vi "pmu_Compute Phasor Indexes.vi"(8 "error in (no error)":errorcluster, 10 "physical channels":T3[](array[typedef]), 11 "phasor channels":T2[](array[typedef]) {"phasor unit scaling" max=16777215 format="%06x"; "phasor unit" items=["Voltage [V]"=0, "Current [A]"=16777216]}) -> (0 "error out":errorcluster, 3 "phasor channel info":T1[](array[typedef]))   [LabVIEW 2011, in "NI_EP_PMU.lvlib"]
uses:
  <vilib>/addons/Electrical Power/PMU/NI_EP_PMU.lvlib
  <vilib>/addons/Electrical Power/PMU/Common/Controls/pmu_Physical Channel.ctl
  <vilib>/addons/Electrical Power/PMU/Common/Controls/pmu_Channel Phase.ctl
  <vilib>/addons/Electrical Power/PMU/Common/Controls/pmu_Phasor Channel.ctl
  <vilib>/addons/Electrical Power/PMU/Common/Controls/pmu_Phasor Channel Info.ctl
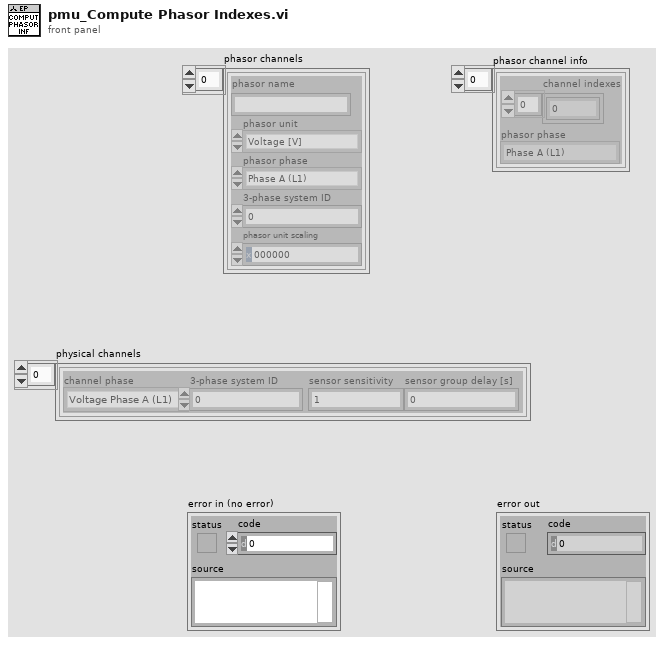
[diagram p1: front panel]
types:
  T1 = typedef "NI_EP_PMU.lvlib/pmu_Phasor Channel Info.ctl" = cluster{"channel indexes":i32[], "phasor phase":enum16{"Phase A (L1)", "Phase B (L2)", "Phase C (L3)", "Phase N", "Positive sequence", "Negative sequence", "Zero sequence"}}
  T2 = typedef "NI_EP_PMU.lvlib/pmu_Phasor Channel.ctl" = cluster{"phasor name":string, "phasor unit":u32, "phasor phase":enum16{"Phase A (L1)", "Phase B (L2)", "Phase C (L3)", "Phase N", "Positive sequence", "Negative sequence", "Zero sequence"}, "3-phase system ID":u8, "phasor unit scaling":u32}
  T3 = typedef "NI_EP_PMU.lvlib/pmu_Physical Channel.ctl" = cluster{"channel phase":T4, "3-phase system ID":u8, "sensor sensitivity":dbl, "sensor group delay [s]":dbl}
  T4 = typedef "NI_EP_PMU.lvlib/pmu_Channel Phase.ctl" = enum16{"Voltage Phase A (L1)", "Voltage Phase B (L2)", "Voltage Phase C (L3)", "Voltage Phase N (Neutral)", "Current Phase A (L1)", "Current Phase B (L2)", "Current Phase C (L3)", "Current Phase N (Neutral)"}
  T5 = cluster{"3-phase system ID":u8, "channel phase":T4}
  T6 = enum16{"Phase A (L1)", "Phase B (L2)", "Phase C (L3)", "Phase N", "Positive sequence", "Negative sequence", "Zero sequence"}
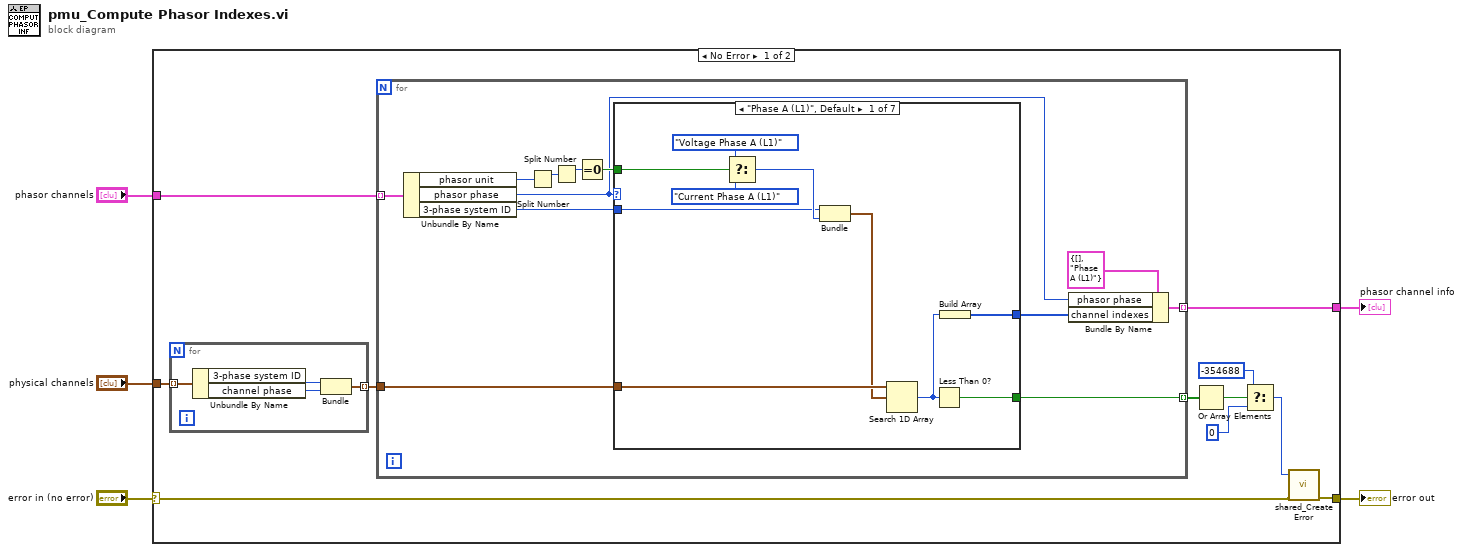
[diagram p0: block diagram]
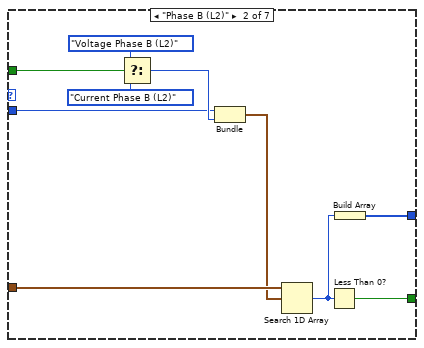
[diagram p2: hidden frame]
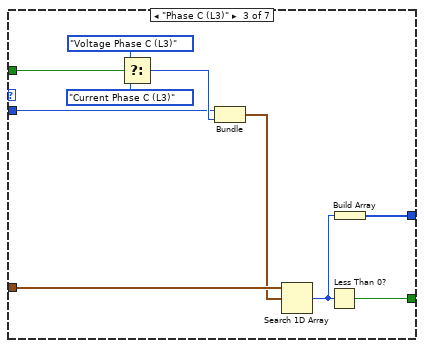
[diagram p3: hidden frame]
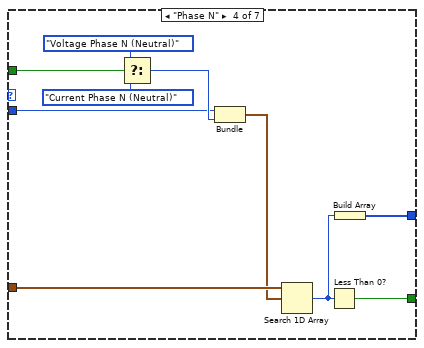
[diagram p4: hidden frame]
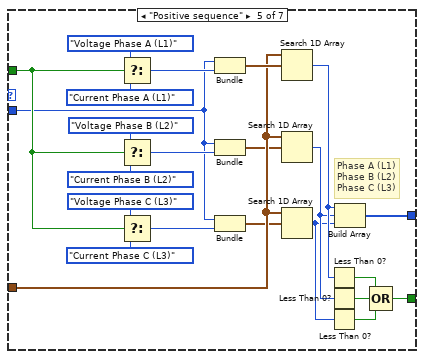
[diagram p5: hidden frame]
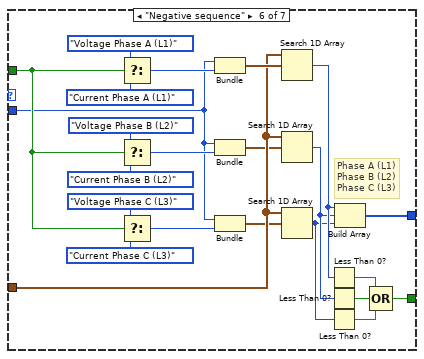
[diagram p6: hidden frame]
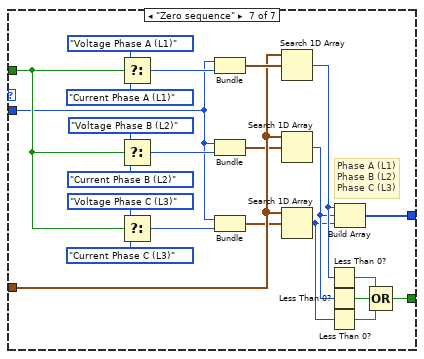
[diagram p7: hidden frame]
diagram:
  n1 = case shown="No Error" "error in (no error)" {
    selector: "error in (no error)" -> [w7 w142]
    tunnel: "phasor channels" -> [w16 _]
    tunnel: "physical channels" -> [w15 _]
    tunnel: [w6 w142] -> w2
    tunnel: [w11 _] -> w1
    frame No Error {
      n2 = for {
        tunnel: w15 -> [w20] mode=indexing
        tunnel: [w19] -> w14 mode=indexing
        n3 = Unbundle By Name(w20) -> ("3-phase system ID"=w17:u8, "channel phase"=w18:T4)
        n4 = Bundle("3-phase system ID"=w17, "channel phase"=w18) -> (w19:T5)  [unwired: 1 in]
      }
      n5 = for {
        tunnel: w16 -> [w32] mode=indexing
        tunnel: w14 -> [w26]
        tunnel: [w25] -> w13 mode=indexing
        tunnel: [w24] -> w11 mode=indexing
        n6 = Unbundle By Name(w32) -> ("phasor unit"=w29:u32, "phasor phase"=w21:T6, "3-phase system ID"=w28:u8)
        n7 = Split Number(x=w29) -> (hi(x)=w31:u16)  [unwired: 1 out]
        n8 = Split Number(x=w31) -> (hi(x)=w30:u8)  [unwired: 1 out]
        n9 = Equal To 0?(x=w30) -> (x = 0?=w27:bool)
        n10 = case shown="\"Phase A (L1)\", Default" w21 {
          tunnel: w28 -> [w38 w48 w58 w68 w84 w107 w130]
          tunnel: w27 -> [w40 w50 w60 w70 w87 w110 w133]
          tunnel: w26 -> [w37 w47 w57 w67 w83 w106 w129]
          tunnel: [w36 w46 w56 w66 w79 w102 w125] -> w25
          tunnel: [w34 w44 w54 w64 w73 w96 w119] -> w22
          frame "Phase A (L1)", Default {
            n11 = Select(t=pmu_Channel_Phase."Voltage Phase A (L1)" ("channel phase"), s=w40, f=pmu_Channel_Phase."Current Phase A (L1)" ("channel phase")) -> (s? t:f=w39:T4)
            n12 = Bundle("3-phase system ID"=w38, "channel phase"=w39) -> (w35:T5)  [unwired: 1 in]
            n13 = Search 1D Array(1D array=w37, element=w35) -> (index of element=w33:i32)  [unwired: 1 in]
            n14 = Less Than 0?(x=w33) -> (x < 0?=w36:bool)
            n15 = Build Array(w33) -> (w34:i32[])
          }
          frame "Phase B (L2)" {
            n16 = Select(t=pmu_Channel_Phase."Voltage Phase B (L2)" ("channel phase"), s=w50, f=pmu_Channel_Phase."Current Phase B (L2)" ("channel phase")) -> (s? t:f=w49:T4)
            n17 = Bundle("3-phase system ID"=w48, "channel phase"=w49) -> (w45:T5)  [unwired: 1 in]
            n18 = Search 1D Array(1D array=w47, element=w45) -> (index of element=w43:i32)  [unwired: 1 in]
            n19 = Less Than 0?(x=w43) -> (x < 0?=w46:bool)
            n20 = Build Array(w43) -> (w44:i32[])
          }
          frame "Phase C (L3)" {
            n21 = Select(t=pmu_Channel_Phase."Voltage Phase C (L3)" ("channel phase"), s=w60, f=pmu_Channel_Phase."Current Phase C (L3)" ("channel phase")) -> (s? t:f=w59:T4)
            n22 = Bundle("3-phase system ID"=w58, "channel phase"=w59) -> (w55:T5)  [unwired: 1 in]
            n23 = Search 1D Array(1D array=w57, element=w55) -> (index of element=w53:i32)  [unwired: 1 in]
            n24 = Less Than 0?(x=w53) -> (x < 0?=w56:bool)
            n25 = Build Array(w53) -> (w54:i32[])
          }
          frame "Phase N" {
            n26 = Select(t=pmu_Channel_Phase."Voltage Phase N (Neutral)" ("channel phase"), s=w70, f=pmu_Channel_Phase."Current Phase N (Neutral)" ("channel phase")) -> (s? t:f=w69:T4)
            n27 = Bundle("3-phase system ID"=w68, "channel phase"=w69) -> (w65:T5)  [unwired: 1 in]
            n28 = Search 1D Array(1D array=w67, element=w65) -> (index of element=w63:i32)  [unwired: 1 in]
            n29 = Less Than 0?(x=w63) -> (x < 0?=w66:bool)
            n30 = Build Array(w63) -> (w64:i32[])
          }
          frame "Positive sequence" {
            # "Phase A (L1)\nPhase B (L2)\nPhase C (L3)"
            n31 = Select(t=pmu_Channel_Phase."Voltage Phase A (L1)" ("channel phase"), s=w87, f=pmu_Channel_Phase."Current Phase A (L1)" ("channel phase")) -> (s? t:f=w93:T4)
            n32 = Select(t=pmu_Channel_Phase."Voltage Phase B (L2)" ("channel phase"), s=w87, f=pmu_Channel_Phase."Current Phase B (L2)" ("channel phase")) -> (s? t:f=w86:T4)
            n33 = Select(t=pmu_Channel_Phase."Voltage Phase C (L3)" ("channel phase"), s=w87, f=pmu_Channel_Phase."Current Phase C (L3)" ("channel phase")) -> (s? t:f=w85:T4)
            n34 = Bundle("3-phase system ID"=w84, "channel phase"=w93) -> (w92:T5)  [unwired: 1 in]
            n35 = Bundle("3-phase system ID"=w84, "channel phase"=w86) -> (w81:T5)  [unwired: 1 in]
            n36 = Bundle("3-phase system ID"=w84, "channel phase"=w85) -> (w82:T5)  [unwired: 1 in]
            n37 = Search 1D Array(1D array=w83, element=w92) -> (index of element=w76:i32)  [unwired: 1 in]
            n38 = Search 1D Array(1D array=w83, element=w81) -> (index of element=w75:i32)  [unwired: 1 in]
            n39 = Search 1D Array(1D array=w83, element=w82) -> (index of element=w74:i32)  [unwired: 1 in]
            n40 = Less Than 0?(x=w76) -> (x < 0?=w80:bool)
            n41 = Less Than 0?(x=w75) -> (x < 0?=w78:bool)
            n42 = Less Than 0?(x=w74) -> (x < 0?=w77:bool)
            n43 = Build Array(w76, w75, w74) -> (w73:i32[])
            n44 = Compound Arithmetic op=OR(w80, w78, w77) -> (w79:bool)
          }
          frame "Negative sequence" {
            # "Phase A (L1)\nPhase B (L2)\nPhase C (L3)"
            n45 = Select(t=pmu_Channel_Phase."Voltage Phase A (L1)" ("channel phase"), s=w110, f=pmu_Channel_Phase."Current Phase A (L1)" ("channel phase")) -> (s? t:f=w116:T4)
            n46 = Select(t=pmu_Channel_Phase."Voltage Phase B (L2)" ("channel phase"), s=w110, f=pmu_Channel_Phase."Current Phase B (L2)" ("channel phase")) -> (s? t:f=w109:T4)
            n47 = Select(t=pmu_Channel_Phase."Voltage Phase C (L3)" ("channel phase"), s=w110, f=pmu_Channel_Phase."Current Phase C (L3)" ("channel phase")) -> (s? t:f=w108:T4)
            n48 = Bundle("3-phase system ID"=w107, "channel phase"=w116) -> (w115:T5)  [unwired: 1 in]
            n49 = Bundle("3-phase system ID"=w107, "channel phase"=w109) -> (w104:T5)  [unwired: 1 in]
            n50 = Bundle("3-phase system ID"=w107, "channel phase"=w108) -> (w105:T5)  [unwired: 1 in]
            n51 = Search 1D Array(1D array=w106, element=w115) -> (index of element=w99:i32)  [unwired: 1 in]
            n52 = Search 1D Array(1D array=w106, element=w104) -> (index of element=w98:i32)  [unwired: 1 in]
            n53 = Search 1D Array(1D array=w106, element=w105) -> (index of element=w97:i32)  [unwired: 1 in]
            n54 = Less Than 0?(x=w99) -> (x < 0?=w103:bool)
            n55 = Less Than 0?(x=w98) -> (x < 0?=w101:bool)
            n56 = Less Than 0?(x=w97) -> (x < 0?=w100:bool)
            n57 = Build Array(w99, w98, w97) -> (w96:i32[])
            n58 = Compound Arithmetic op=OR(w103, w101, w100) -> (w102:bool)
          }
          frame "Zero sequence" {
            # "Phase A (L1)\nPhase B (L2)\nPhase C (L3)"
            n59 = Select(t=pmu_Channel_Phase."Voltage Phase A (L1)" ("channel phase"), s=w133, f=pmu_Channel_Phase."Current Phase A (L1)" ("channel phase")) -> (s? t:f=w139:T4)
            n60 = Select(t=pmu_Channel_Phase."Voltage Phase B (L2)" ("channel phase"), s=w133, f=pmu_Channel_Phase."Current Phase B (L2)" ("channel phase")) -> (s? t:f=w132:T4)
            n61 = Select(t=pmu_Channel_Phase."Voltage Phase C (L3)" ("channel phase"), s=w133, f=pmu_Channel_Phase."Current Phase C (L3)" ("channel phase")) -> (s? t:f=w131:T4)
            n62 = Bundle("3-phase system ID"=w130, "channel phase"=w139) -> (w138:T5)  [unwired: 1 in]
            n63 = Bundle("3-phase system ID"=w130, "channel phase"=w132) -> (w127:T5)  [unwired: 1 in]
            n64 = Bundle("3-phase system ID"=w130, "channel phase"=w131) -> (w128:T5)  [unwired: 1 in]
            n65 = Search 1D Array(1D array=w129, element=w138) -> (index of element=w122:i32)  [unwired: 1 in]
            n66 = Search 1D Array(1D array=w129, element=w127) -> (index of element=w121:i32)  [unwired: 1 in]
            n67 = Search 1D Array(1D array=w129, element=w128) -> (index of element=w120:i32)  [unwired: 1 in]
            n68 = Less Than 0?(x=w122) -> (x < 0?=w126:bool)
            n69 = Less Than 0?(x=w121) -> (x < 0?=w124:bool)
            n70 = Less Than 0?(x=w120) -> (x < 0?=w123:bool)
            n71 = Build Array(w122, w121, w120) -> (w119:i32[])
            n72 = Compound Arithmetic op=OR(w126, w124, w123) -> (w125:bool)
          }
        }
        n73 = Bundle By Name(cluster=T1 {"channel indexes"=[], "phasor phase"=enum."Phase A (L1)"} ("phasor index"), "phasor phase"=w21, "channel indexes"=w22) -> (w24:T1)
      }
      n74 = Or Array Elements(Boolean array=w13) -> (logical OR=w12:bool)
      n75 = Select(t=-354688 ("error code (0)"), s=w12, f=0 ("error code (0)")) -> (s? t:f=w8:i32)
      n76 = call <vilib>:"shared_Create Error.vi"("error in (no error)"=w7, "error code (0)"=w8) -> ("error out"=w6:errorcluster)  [unwired: 9 in]
    }
    frame Error {
    }
  }
  "error out" <- w2
  "phasor channel info" <- w1
